vi "Temp conversion using case structures.vi"() -> ()   [LabVIEW 2018]
panel:
  out "Celsius":dbl(slide) scale=0.0..400.0
  out "Celsius":dbl
  out "Kelvin":dbl
  out "Fahrenheit":dbl
  out "Kelvin":dbl(slide) scale=0.0..400.0
  in  "Fahrenheit":dbl(slide) scale=0.0..400.0
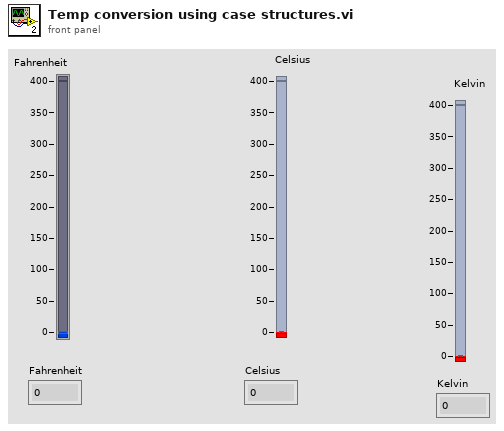
[diagram p1: front panel]
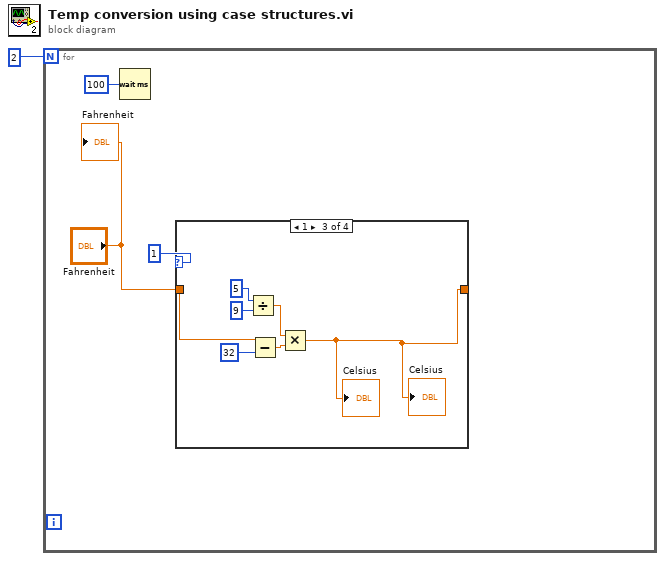
[diagram p0: block diagram]
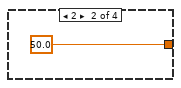
[diagram p3: hidden frame]
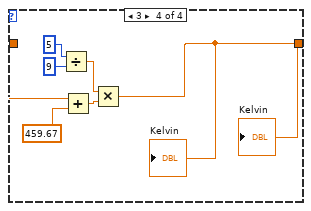
[diagram p4: hidden frame]
diagram:
  n1 = for {
    N: 2 -> [_]
    n2 = Wait (ms)(milliseconds to wait=100) -> ()  [unwired: 1 out]
    n3 = case shown="1" 1 {
      tunnel: "Fahrenheit" -> [w5 _ w13 w15]
      tunnel: [w5 50.0 ("Fahrenheit") w7 w14] -> _
      frame 0, Default {
      }
      frame 2 {
      }
      frame 1 {
        n4 = Divide(x=5, y=9) -> (x/y=w12:dbl)
        n5 = Subtract(x=w13, y=32) -> (x-y=w11:dbl)
        n6 = Multiply(x=w12, y=w11) -> (x*y=w7:dbl)
        "Celsius" <- w7
        "Celsius" <- w7
      }
      frame 3 {
        n7 = Divide(x=5, y=9) -> (x/y=w20:dbl)
        n8 = Add(x=w15, y=459.67) -> (x+y=w19:dbl)
        n9 = Multiply(x=w20, y=w19) -> (x*y=w14:dbl)
        "Kelvin" <- w14
        "Kelvin" <- w14
      }
    }
    "Fahrenheit" <- "Fahrenheit"
  }
